vi "get_output_channel.vi"(8 "error in (no error)":errorcluster, 11 "heat_board_control in":refnum<class "heat_board_control.lvclass">) -> (0 "error out":errorcluster, 2 "physical channel":refnum<k21>="Dev0/Ao0", 3 "heat_board_control out":refnum<class "heat_board_control.lvclass">)   [LabVIEW 2015, in "heat_board_control.lvclass"]
uses:
  heat_board_control.lvclass
  heat_board_control.lvclass/heat_board_control.ctl
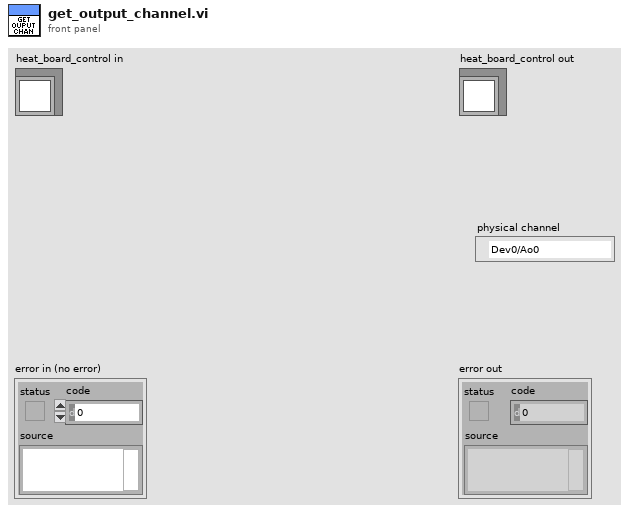
[diagram p1: front panel]
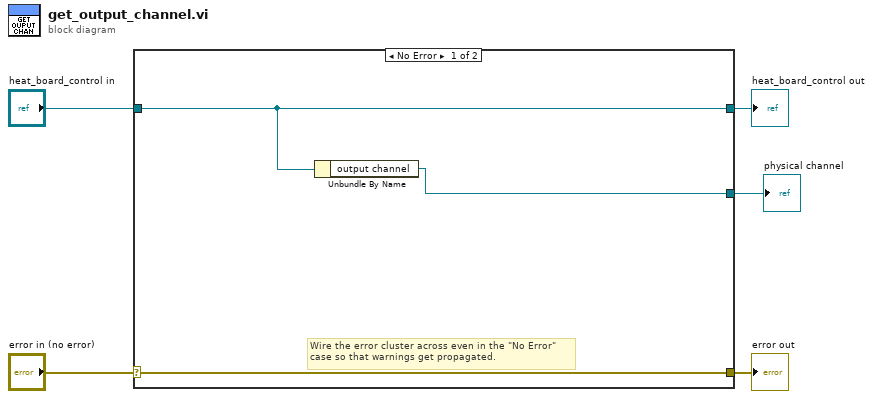
[diagram p0: block diagram]
diagram:
  n1 = case shown="No Error" "error in (no error)" {
    selector: "error in (no error)" -> [w8 w10]
    tunnel: [w8 w10] -> w4
    tunnel: [w7 w9] -> w2
    tunnel: "heat_board_control in" -> [w7 w9]
    tunnel: [w6 _] -> w1
    frame No Error {
      # "Wire the error cluster across even in the \"No Error\"\ncase so that warnings get propagated."
      n2 = Unbundle By Name(w7) -> ("output channel"=w6:refnum<k21>)
    }
    frame Error {
    }
  }
  "error out" <- w4
  "heat_board_control out" <- w2
  "physical channel" <- w1
